vi "cburen_Gen_Test_Single_Cell.vi"() -> ()   [LabVIEW 2020]
panel:
  in  "Output Safety":T1
  in  "filepath":path
  in  "Batteryname":string
  in  "Starting Cycle":i32
  out "PS error out":errorcluster
  out "PS VIS resource name out":refnum<visa-resource-name>
  out "data task error out":errorcluster
  out "data task out":refnum<k21>
  in  "Charge Current Cutoff":dbl
  in  "Charge Current Setpoint 2":dbl format="%#.6g"
  in  "charge Voltage Setpoint  2":dbl format="%#.6g"
  in  "Wait time":dbl
  in  "Discharge Current Cutoff":dbl
  in  "Discharge Current Setpoint":dbl format="%#.6g"
  in  "Discharge Voltage Setpoint":dbl format="%#.6g"
  in  "NHR VISA":refnum<visa-resource-name>
  in  "NHR error in":errorcluster
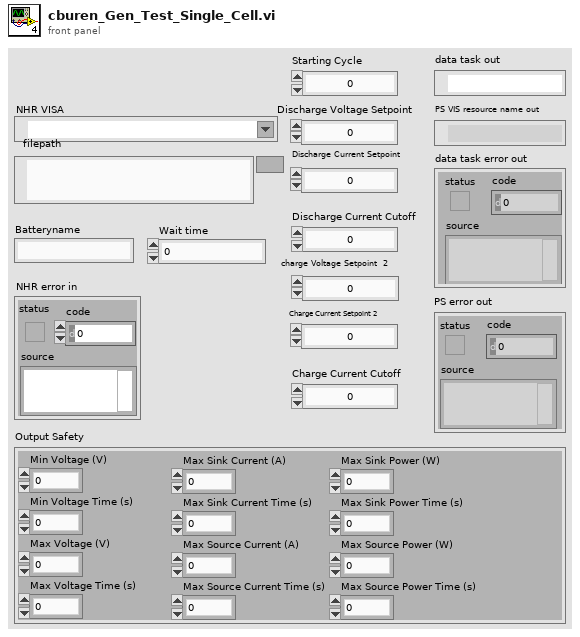
[diagram p1: front panel]
types:
  T1 = cluster{"Min Voltage (V)":dbl, "Min Voltage Time (s)":dbl, "Max Voltage (V)":dbl, "Max Voltage Time (s)":dbl, "Max Sink Current (A)":dbl, "Max Sink Current Time (s)":dbl, "Max Source Current (A)":dbl, "Max Source Current Time (s)":dbl, "Max Sink Power (W)":dbl, "Max Sink Power Time (s)":dbl, "Max Source Power (W)":dbl, "Max Source Power Time (s)":dbl}
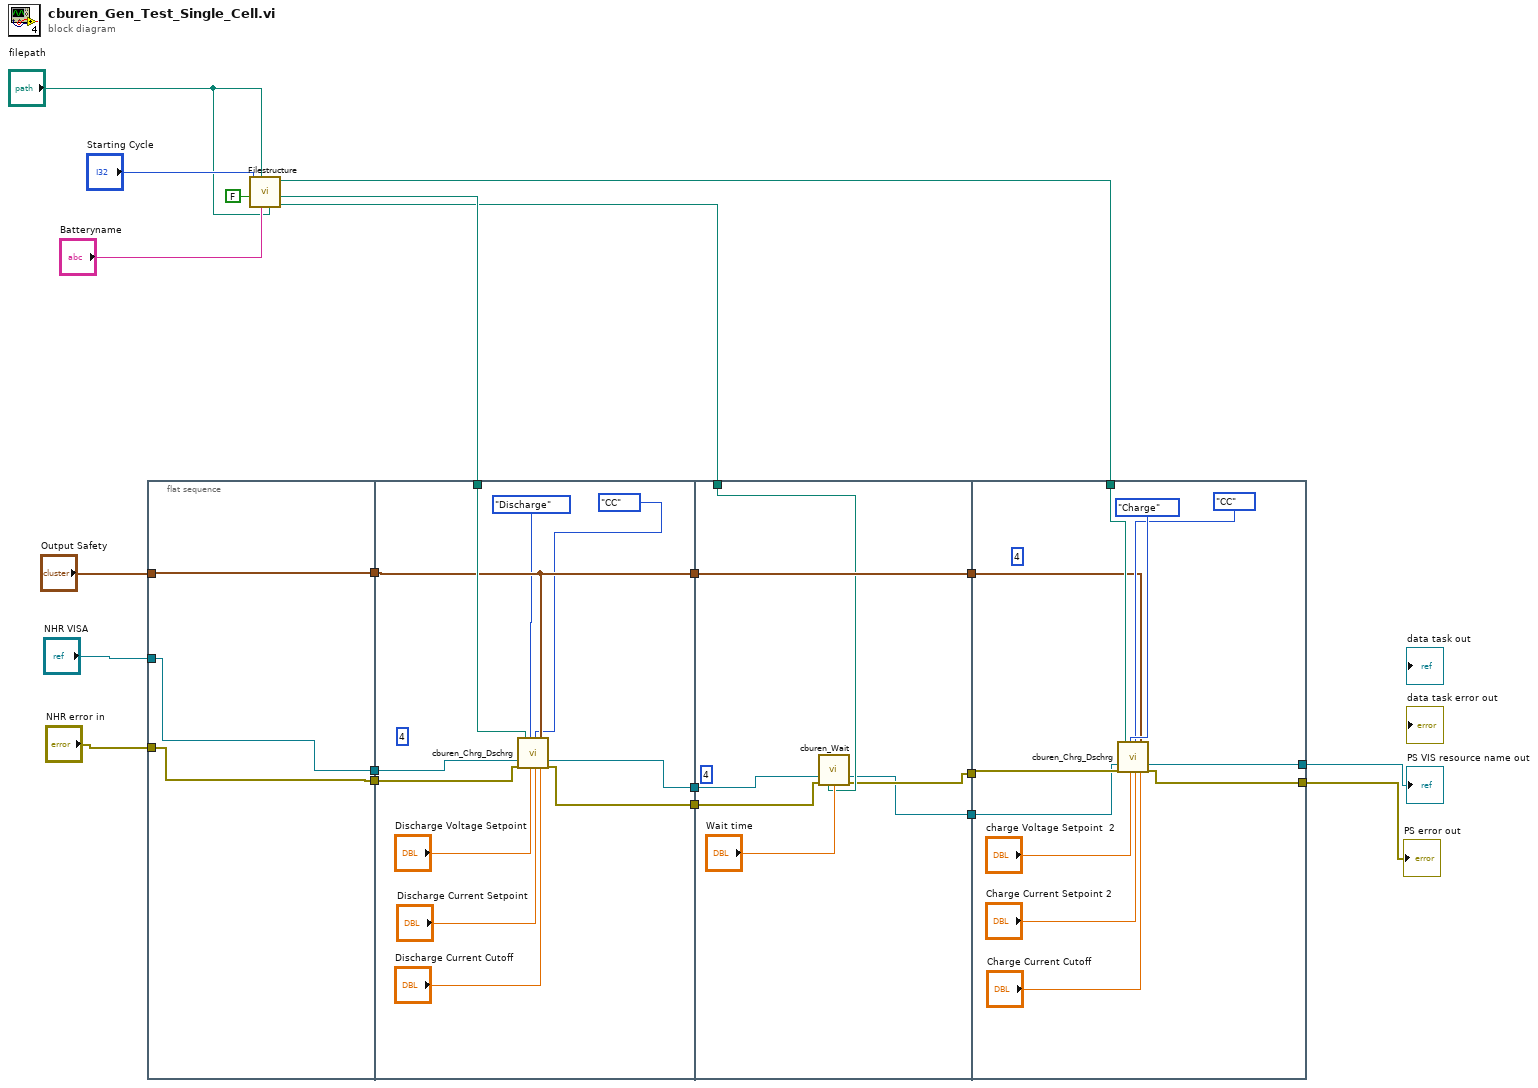
[diagram p0: block diagram]
diagram:
  n1 = flat-sequence {
    tunnel: "NHR error in" -> [w23]
    tunnel: "NHR VISA" -> [w24]
    tunnel: [w24] -> w19
    tunnel: [w23] -> w18
    tunnel: "Output Safety" -> [w22]
    tunnel: [w22] -> w8
    tunnel: w19 -> [w33]
    tunnel: w18 -> [w32]
    tunnel: w12 -> [w35]
    tunnel: w8 -> [w34]
    tunnel: [w34] -> w7
    tunnel: [w28] -> w4
    tunnel: [w27] -> w3
    tunnel: [w37] -> w17
    tunnel: [w36] -> w16
    tunnel: w11 -> [w38]
    tunnel: w7 -> [w42]
    tunnel: [w42] -> w6
    tunnel: w4 -> [w41]
    tunnel: w3 -> [w40]
    tunnel: w17 -> [w53]
    tunnel: w16 -> [w52]
    tunnel: w10 -> [w51]
    tunnel: w6 -> [w48]
    tunnel: [w44] -> w1
    tunnel: [w43] -> w2
    frame #0 {
    }
    frame #1 {
      (unwired) 4 ("#DAQ outputs (1-13)")
      n2 = call "cburen_Chrg_Dschrg.vi"("PS VISA in"=w33, "PS error in"=w32, "DischargeCyclePath"=w35, "Charge/discharge"=enum8{"Charge", "Discharge"}."Discharge", "Charge/Discharge Voltage Setpoint"="Discharge Voltage Setpoint", "CC or CCCV"=enum16{"CC", "CCCV"}."CC", "Current Setpoint"="Discharge Current Setpoint", "Output Safety"=w34, "Current Cutoff"="Discharge Current Cutoff") -> ("PS VIS resource name out"=w27:refnum<visa-resource-name>, "PS error out"=w28:errorcluster)  [unwired: 9 in]
    }
    frame #2 {
      (unwired) 4 ("#DAQ outputs (1-13)")
      n3 = call "cburen_Wait.vi"("PS VISA in"=w40, "PS error in"=w41, "Wait Filepath"=w38, "Wait time"="Wait time") -> ("PS Visa Out"=w36:refnum<visa-resource-name>, "PS error out"=w37:errorcluster)  [unwired: 10 in]
    }
    frame #3 {
      (unwired) 4 ("#DAQ outputs (1-13)")
      n4 = call "cburen_Chrg_Dschrg.vi"("PS VISA in"=w52, "PS error in"=w53, "DischargeCyclePath"=w51, "Charge/discharge"=enum8{"Charge", "Discharge"}."Charge", "Charge/Discharge Voltage Setpoint"="charge Voltage Setpoint  2", "CC or CCCV"=enum16{"CC", "CCCV"}."CC", "Current Setpoint"="Charge Current Setpoint 2", "Output Safety"=w48, "Current Cutoff"="Charge Current Cutoff") -> ("PS VIS resource name out"=w44:refnum<visa-resource-name>, "PS error out"=w43:errorcluster)  [unwired: 9 in]
    }
  }
  n5 = call "Filestructure.vi"("Discharge filepath"="filepath", "Batteryname"="Batteryname", "Charge filepath"="filepath", "In for loop"=FALSE, "Starting Cycle"="Starting Cycle") -> ("DischargeWaitPath"=w11:path, "DischargeCyclePath"=w12:path, "ChargeCyclePath"=w10:path)  [unwired: 2 in, 2 out]
  "PS error out" <- w2
  "PS VIS resource name out" <- w1
